vi "Agilent PSG MXG Series Configure Frequency Power.vi"() -> ()   [LabVIEW 2009]
doc: "This example shows how to configure the frequency and power of the output signal."
uses:
  Agilent PSG MXG Series.lvlib
panel:
  in  "VISA resource name":refnum<visa-resource-name>
  in  "ALC Level (1 dB)":dbl=1.0
  in  "Power Offset (0 dB)":dbl
  in  "Power Reference (0 dBm)":dbl
  in  "Power (-130 dBm)":dbl=-130.0
  in  "Attenuation Level (115 dB)":dbl=115.0
  in  "Attenuator Auto Mode (T:Enable)":bool=TRUE
  in  "Offset Frequency (0 Hz)":dbl
  in  "Reference Frequency (0 Hz)":dbl
  in  "Frequency (100 kHz)":dbl=100000.0
  # "(c) 2009 National Instruments.  ALL RIGHTS RESERVED."
  # "Note: Attenuation Level and ALC Level are valid only when\nAttenuator Auto Mode is FALSE.\nAnd the output power is ALC Level minus Attenuation Level."
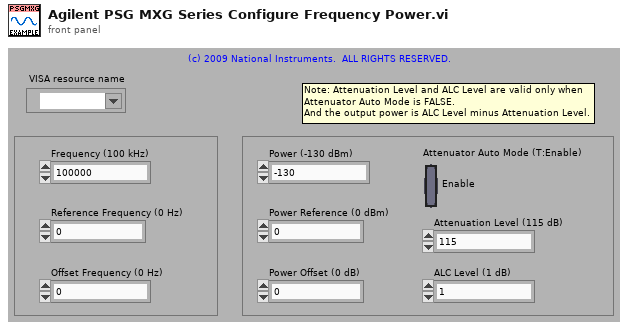
[diagram p1: front panel]
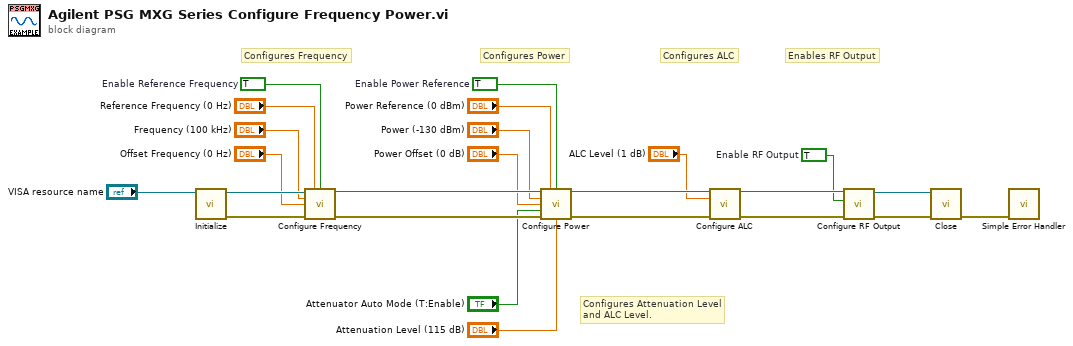
[diagram p0: block diagram]
diagram:
  w1 = TRUE  # Enable RF Output
  w6 = TRUE  # Enable Power Reference
  w9 = TRUE  # Enable Reference Frequency
  # "Configures Attenuation Level\nand ALC Level."
  # "Enables RF Output"
  # "Configures ALC"
  # "Configures Power"
  # "Configures Frequency"
  n1 = call "Initialize.vi"("VISA resource name"="VISA resource name") -> ("error out"=w23:errorcluster, "VISA resource name out"=w24:refnum<visa-resource-name>)  [unwired: 3 in, 6 out]
  n2 = call "Configure Frequency.vi"("VISA resource name"=w24, "Reference Frequency (0 Hz)"="Reference Frequency (0 Hz)", "Enable Reference Frequency (F:Disable)"=w9, "Frequency (100 kHz)"="Frequency (100 kHz)", "Offset Frequency (0 Hz)"="Offset Frequency (0 Hz)", "error in (no error)"=w23) -> ("VISA resource name out"=w22:refnum<visa-resource-name>, "error out"=w21:errorcluster)  [unwired: 3 in, 5 out]
  n3 = call "Configure Power.vi"("VISA resource name"=w22, "Power Reference (0 dBm)"="Power Reference (0 dBm)", "Enable Power Reference (F:Disable)"=w6, "Power (-130 dBm)"="Power (-130 dBm)", "Power Offset (0 dB)"="Power Offset (0 dB)", "Attenuator Auto Mode (T:Enable)"="Attenuator Auto Mode (T:Enable)", "error in (no error)"=w21, "Attenuation Level (115 dB)"="Attenuation Level (115 dB)") -> ("VISA resource name out"=w20:refnum<visa-resource-name>, "error out"=w19:errorcluster)  [unwired: 2 in, 4 out]
  n4 = call "Configure ALC.vi"("VISA resource name"=w20, "ALC Level (1 dB)"="ALC Level (1 dB)", "error in (no error)"=w19) -> ("VISA resource name out"=w17:refnum<visa-resource-name>, "error out"=w16:errorcluster)  [unwired: 5 in, 6 out]
  n5 = call "Configure RF Output.vi"("error in (no error)"=w16, "Enable RF Output (F:Disable)"=w1, "VISA resource name"=w17) -> ("error out"=w14:errorcluster, "VISA resource name out"=w15:refnum<visa-resource-name>)  [unwired: 5 in, 2 out]
  n6 = call "Close.vi"("error in (no error)"=w14, "VISA resource name"=w15) -> ("error out"=w18:errorcluster)  [unwired: 9 out]
  n7 = call <vilib>:"Simple Error Handler.vi"("error in (no error)"=w18) -> ()  [unwired: 1 in, 8 out]
